vi "convert old sequence step def to latest_bool.vi"(8 "error in":errorcluster, 11 "data string":string) -> (0 "error out":errorcluster, 3 "RSLinx String Cluster out":T1={"Data Boolean"=FALSE, "PLC Path and Tag"={"Tag Name"="", "Network Path"="", "use opc"=FALSE, "DataSocket Reference"={"CWDSLib._DCWDataSocket"=refnum, "CWDSLib._DCWData"=refnum, "OnDataUpdated"=0, "OnStatusUpdated"=0}}, "Error No."=157, "timeout (ms)"=1000, "Continue on Fail for Red-Rabbit"=FALSE} {"PLC Path and Tag"."DataSocket Reference"."OnStatusUpdated" format="%.0x"; "PLC Path and Tag"."DataSocket Reference"."OnDataUpdated" format="%.0x"})   [LabVIEW 2018]
uses:
  type defs/RSLinx Boolean Cluster.ctl
  type defs/plc path and tag.ctl
  <vilib>/Platform/dataskt.llb/DataSocket Reference Type.ctl
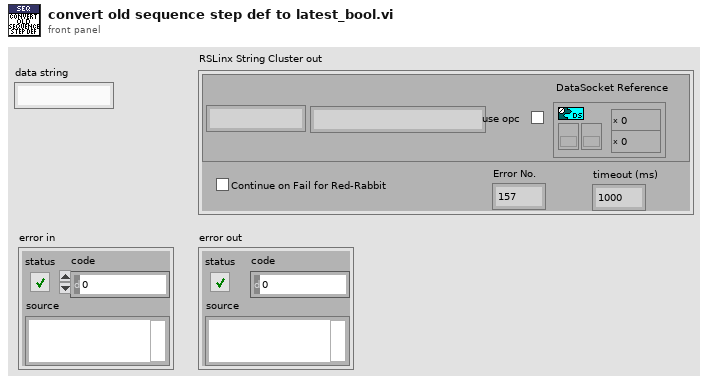
[diagram p1: front panel]
types:
  T1 = typedef "RSLinx Boolean Cluster.ctl" = cluster{"Data Boolean":bool, "PLC Path and Tag":T2, "Error No.":u16, "timeout (ms)":i32, "Continue on Fail for Red-Rabbit":bool}
  T2 = typedef "plc path and tag.ctl" = cluster{"Tag Name":string, "Network Path":string, "use opc":bool, "DataSocket Reference":T3}
  T3 = typedef "DataSocket Reference Type.ctl" = cluster{"CWDSLib._DCWDataSocket":refnum<k7>, "CWDSLib._DCWData":refnum<k7>, "OnDataUpdated":u32, "OnStatusUpdated":u32}
  T4 = cluster{"Data Boolean":bool, "PLC Path and Tag":cluster{"Tag Name":string, "Network Path":string, "use opc":bool, "DataSocket Reference":cluster{"CWDSLib._DCWDataSocket":refnum<k7>, "CWDSLib._DCWData":refnum<k7>, "OnDataUpdated":u32, "OnStatusUpdated":u32}}, "Error No.":u16, "timeout (ms)":i32}
  T5 = cluster{"Data Boolean":bool, "PLC Path and Tag":cluster{"Tag Name":string, "Network Path":string, "use opc":bool, "DataSocket Reference":cluster{"CWDSLib._DCWDataSocket":refnum<k7>, "CWDSLib._DCWData":refnum<k7>, "OnDataUpdated":u32, "OnStatusUpdated":u32}}, "Error No.":u16}
  T6 = cluster{"Tag Name":string, "Network Path":string, "use opc":bool, "DataSocket Reference":cluster{"CWDSLib._DCWDataSocket":refnum<k7>, "CWDSLib._DCWData":refnum<k7>, "OnDataUpdated":u32, "OnStatusUpdated":u32}}
  T7 = cluster{"Data Boolean":bool, "PLC Path and Tag":T2}
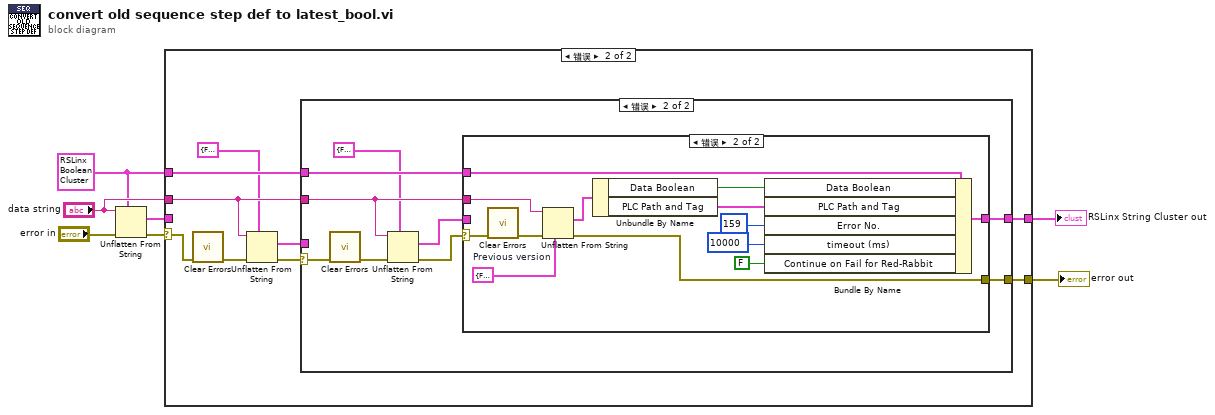
[diagram p0: block diagram]
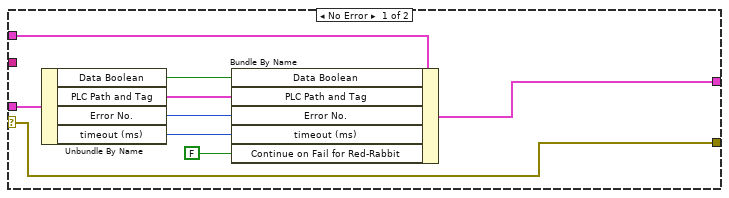
[diagram p3: hidden frame]
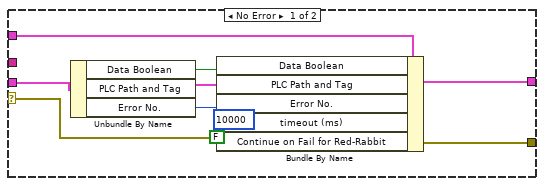
[diagram p4: hidden frame]
diagram:
  w3 = T1 {"Data Boolean"=FALSE, "PLC Path and Tag"={"Tag Name"="", "Network Path"="", "use opc"=FALSE, "DataSocket Reference"={"CWDSLib._DCWDataSocket"=refnum, "CWDSLib._DCWData"=refnum, "OnDataUpdated"=0, "OnStatusUpdated"=0}}, "Error No."=157, "timeout (ms)"=0, "Continue on Fail for Red-Rabbit"=FALSE} ("RSLinx String Cluster in")
  n1 = Unflatten From String(type=w3, binary string="data string", error in (no error)="error in") -> (value=w6:T1, error out=w5:errorcluster)  [unwired: 2 in, 1 out]
  n2 = case shown="错误" w5 {
    selector: w5 -> [w8 w14]
    tunnel: [w9 w17] -> w7
    tunnel: w6 -> [w9 _]
    tunnel: "data string" -> [_ w12]
    tunnel: w3 -> [_ w18]
    tunnel: [w8 w16] -> w1
    frame No Error {
    }
    frame Error {
      n3 = call <vilib>:"Clear Errors.vi"("error in (no error)"=w14) -> ("error out"=w15:errorcluster)  [unwired: 5 in, 1 out]
      n4 = Unflatten From String(type=T4 {"Data Boolean"=FALSE, "PLC Path and Tag"={"Tag Name"="", "Network Path"="", "use opc"=FALSE, "DataSocket Reference"={"CWDSLib._DCWDataSocket"=refnum, "CWDSLib._DCWData"=refnum, "OnDataUpdated"=0, "OnStatusUpdated"=0}}, "Error No."=157, "timeout (ms)"=0} ("RSLinx String Cluster in"), binary string=w12, error in (no error)=w15) -> (value=w10:T4, error out=w13:errorcluster)  [unwired: 2 in, 1 out]
      n5 = case shown="错误" w13 {
        selector: w13 -> [w24 w28]
        tunnel: w18 -> [w26 w36]
        tunnel: [w25 w35] -> w17
        tunnel: [w24 w34] -> w16
        tunnel: w12 -> [_ w32]
        tunnel: w10 -> [w27 _]
        frame No Error {
          n6 = Unbundle By Name(w27) -> ("Data Boolean"=w23:bool, "PLC Path and Tag"=w22:T6, "Error No."=w21:u16, "timeout (ms)"=w20:i32)
          n7 = Bundle By Name(cluster=w26, "Data Boolean"=w23, "PLC Path and Tag"=w22, "Error No."=w21, "timeout (ms)"=w20, "Continue on Fail for Red-Rabbit"=FALSE ("Failures Dont Stop Sequence for Red-Rabbit")) -> (w25:T1)
        }
        frame Error {
          n8 = call <vilib>:"Clear Errors.vi"("error in (no error)"=w28) -> ("error out"=w33:errorcluster)  [unwired: 5 in, 1 out]
          n9 = Unflatten From String(type=T5 {"Data Boolean"=FALSE, "PLC Path and Tag"={"Tag Name"="", "Network Path"="", "use opc"=FALSE, "DataSocket Reference"={"CWDSLib._DCWDataSocket"=refnum, "CWDSLib._DCWData"=refnum, "OnDataUpdated"=0, "OnStatusUpdated"=0}}, "Error No."=157} ("RSLinx String Cluster in"), binary string=w32, error in (no error)=w33) -> (value=w29:T5, error out=w30:errorcluster)  [unwired: 2 in, 1 out]
          n10 = case shown="错误" w30 {
            selector: w30 -> [w39 w48]
            tunnel: w32 -> [_ w58]
            tunnel: w36 -> [w42 w56]
            tunnel: [w41 w55] -> w35
            tunnel: [w39 w49] -> w34
            tunnel: w29 -> [w40 _]
            frame No Error {
              n11 = Unbundle By Name(w40) -> ("Data Boolean"=w43:bool, "PLC Path and Tag"=w44:T6, "Error No."=w45:u16)
              n12 = Bundle By Name(cluster=w42, "Data Boolean"=w43, "PLC Path and Tag"=w44, "Error No."=w45, "timeout (ms)"=10000, "Continue on Fail for Red-Rabbit"=FALSE) -> (w41:T1)
            }
            frame Error {
              w57 = T7 {"Data Boolean"=FALSE, "PLC Path and Tag"={"Tag Name"="", "Network Path"="", "use opc"=FALSE, "DataSocket Reference"={"CWDSLib._DCWDataSocket"=refnum, "CWDSLib._DCWData"=refnum, "OnDataUpdated"=0, "OnStatusUpdated"=0}}}  # Previous version
              n13 = call <vilib>:"Clear Errors.vi"("error in (no error)"=w48) -> ("error out"=w50:errorcluster)  [unwired: 5 in, 1 out]
              n14 = Unflatten From String(type=w57, binary string=w58, error in (no error)=w50) -> (value=w54:T7, error out=w49:errorcluster)  [unwired: 2 in, 1 out]
              n15 = Unbundle By Name(w54) -> ("Data Boolean"=w53:bool, "PLC Path and Tag"=w52:T2)
              n16 = Bundle By Name(cluster=w56, "Data Boolean"=w53, "PLC Path and Tag"=w52, "Error No."=u16 159, "timeout (ms)"=10000, "Continue on Fail for Red-Rabbit"=FALSE) -> (w55:T1)
            }
          }
        }
      }
    }
  }
  "RSLinx String Cluster out" <- w7
  "error out" <- w1
